vi "类型3一组自动测试.vi"(11 "测试值":u16) -> ()   [LabVIEW 2010]
uses:
  全局量/试验配置信息.vi
panel:
  out "D_IN_3":string[][](table) caption="表格"
  out "结束？":bool
  in  "同步_2":i32
  in  "同步_1":i32
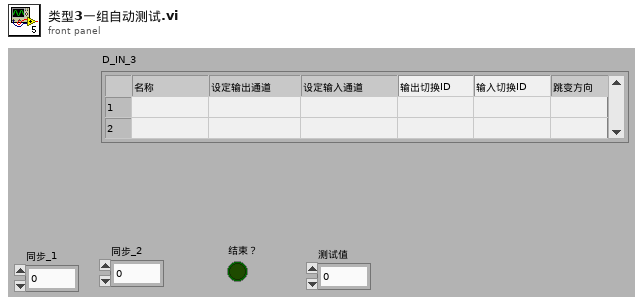
[diagram p1: front panel]
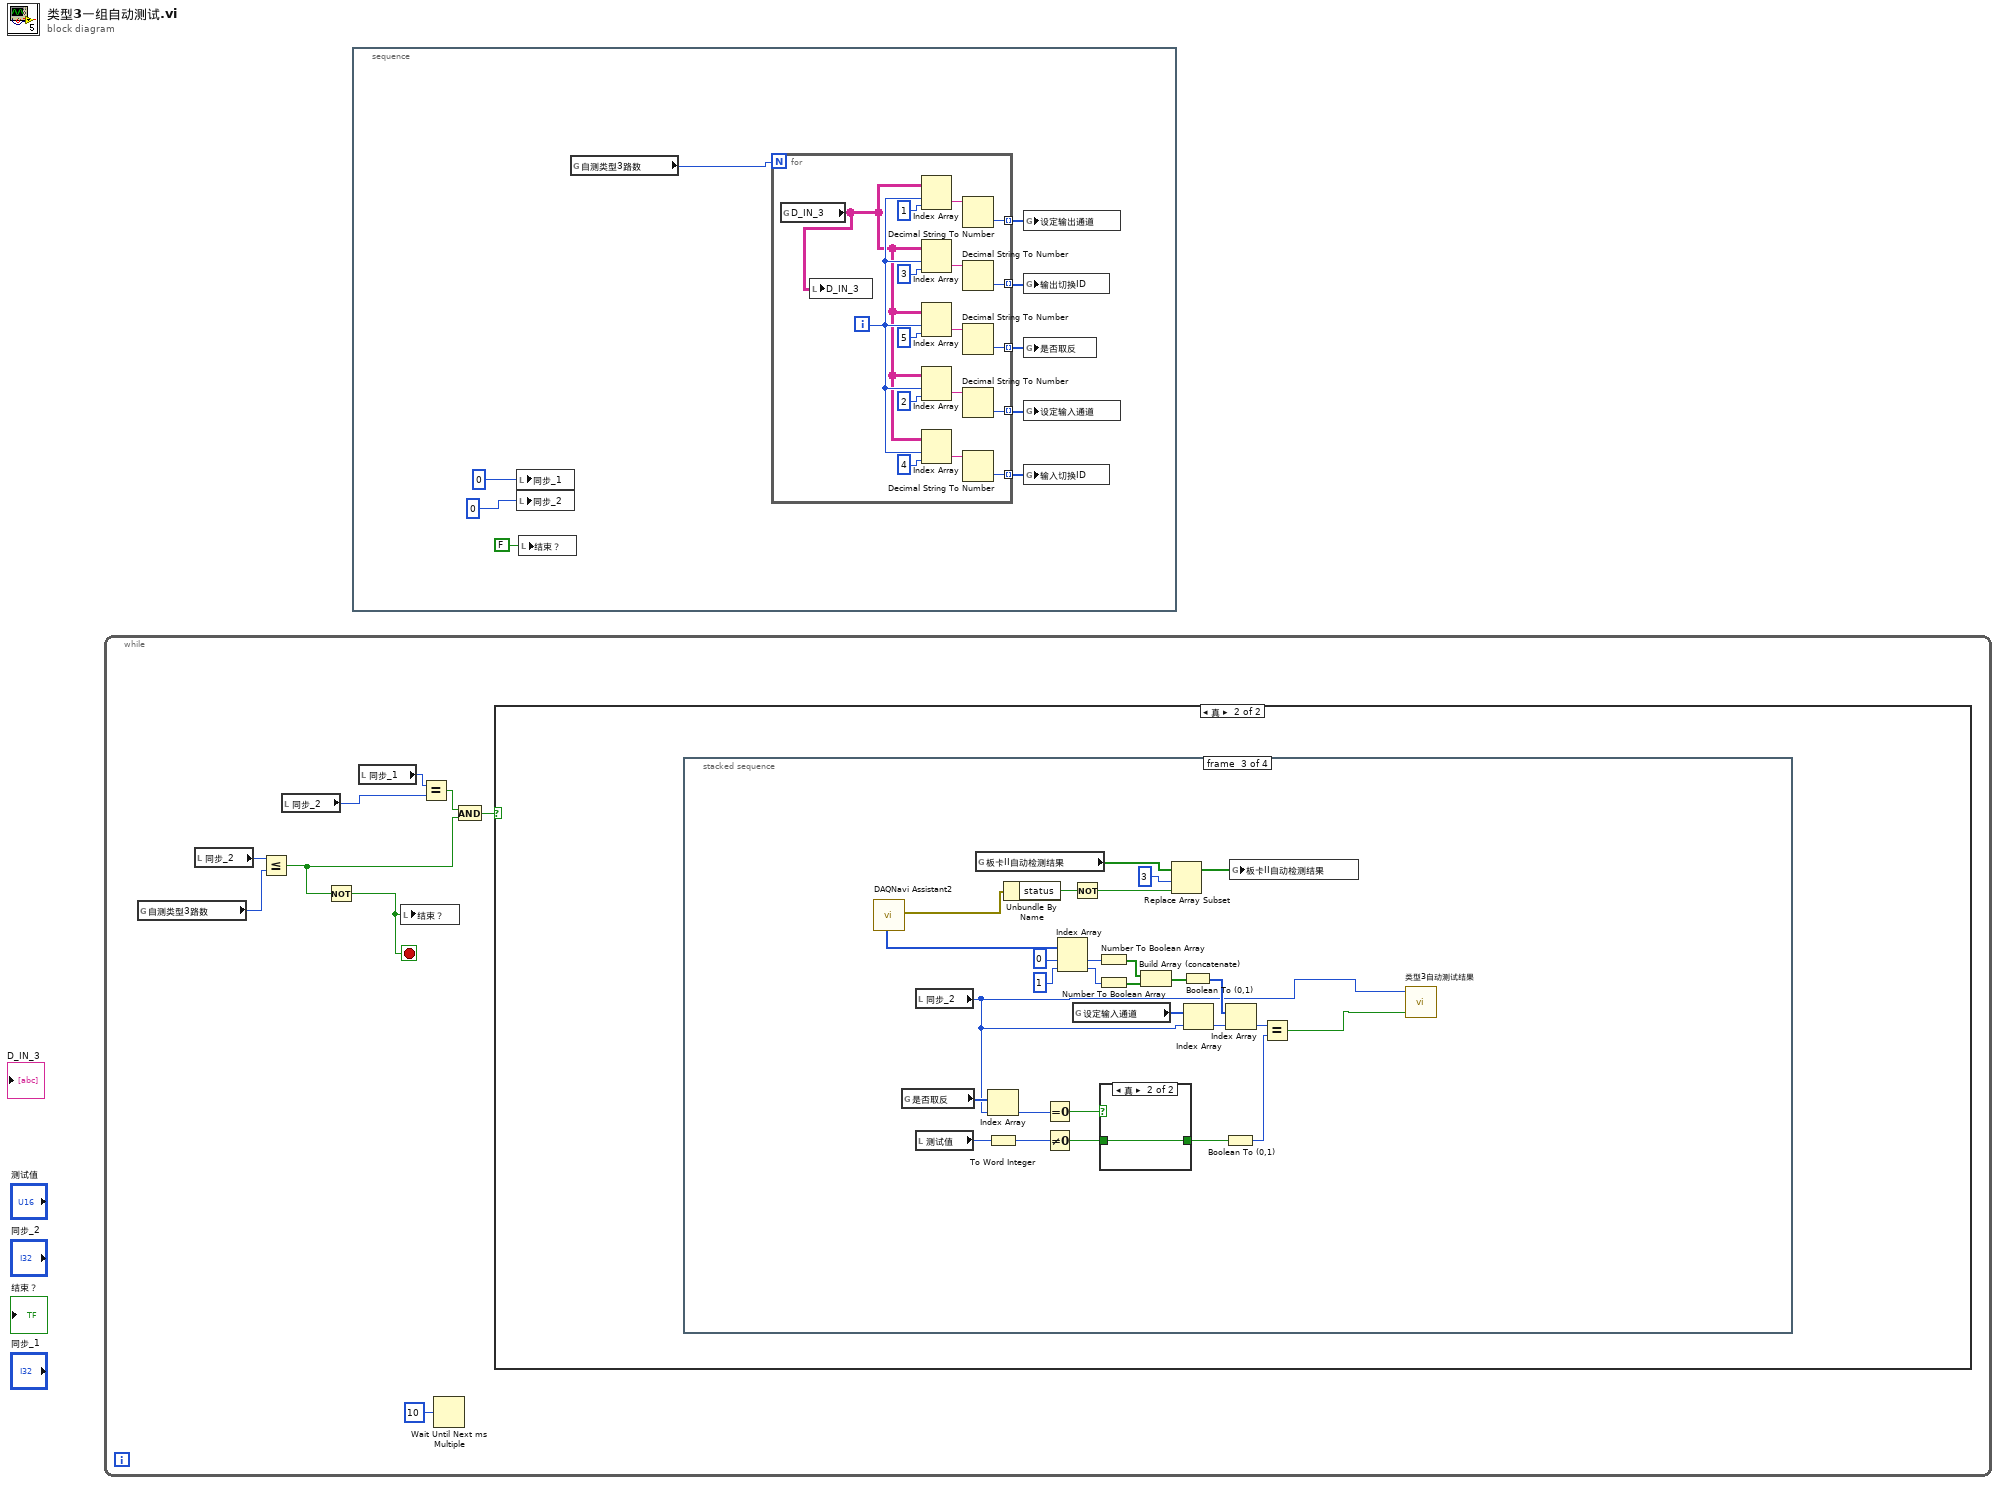
[diagram p0: block diagram]
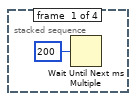
[diagram p3: hidden frame]
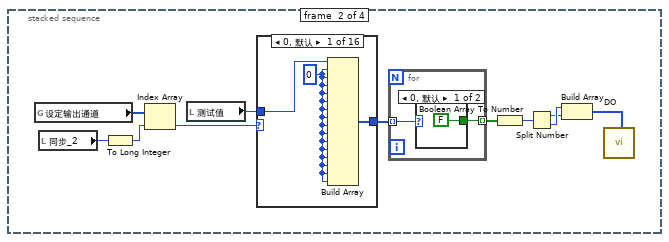
[diagram p4: hidden frame]
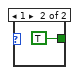
[diagram p5: hidden frame]
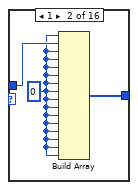
[diagram p6: hidden frame]
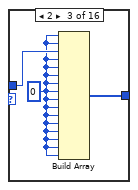
[diagram p7: hidden frame]
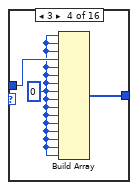
[diagram p8: hidden frame]
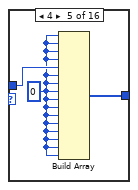
[diagram p9: hidden frame]
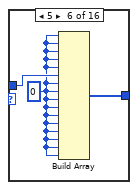
[diagram p10: hidden frame]
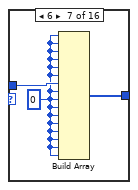
[diagram p11: hidden frame]
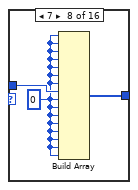
[diagram p12: hidden frame]
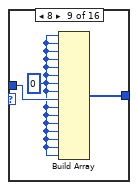
[diagram p13: hidden frame]
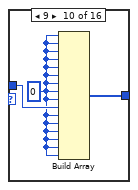
[diagram p14: hidden frame]
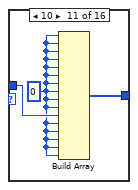
[diagram p15: hidden frame]
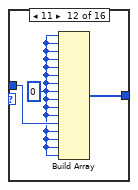
[diagram p16: hidden frame]
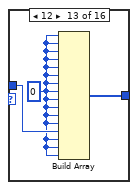
[diagram p17: hidden frame]
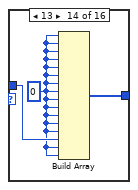
[diagram p18: hidden frame]
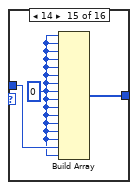
[diagram p19: hidden frame]
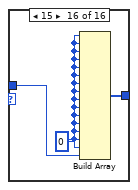
[diagram p20: hidden frame]
diagram:
  n1 = while {
    stop <- w2 stop-if-true
    n2 = global read "试验配置信息.vi" "自测类型3路数"() -> (w1:i32)
    n3 = local read "同步_2"() -> (w4:i32)
    n4 = Less Or Equal?(x=w4, y=w1) -> (x <= y?=w5:bool)
    n5 = local read "同步_2"() -> (w3:i32)
    n6 = Not(x=w5) -> (.not. x?=w2:bool)
    n7 = local read "同步_1"() -> (w8:i32)
    n8 = local write "结束？"(w2) -> ()
    n9 = Equal?(x=w8, y=w3) -> (x = y?=w6:bool)
    n10 = Wait Until Next ms Multiple(millisecond multiple=u32 10 ("毫秒倍数")) -> ()  [unwired: 1 out]
    n11 = And(x=w6, y=w5) -> (x .and. y?=w7:bool)
    n12 = case shown="真" w7 {
      frame False {
      }
      frame True {
        n13 = stacked-sequence {
          frame #0 {
            n14 = Wait Until Next ms Multiple(millisecond multiple=u32 200 ("毫秒倍数")) -> ()  [unwired: 1 out]
          }
          frame #1 {
            n15 = global read "试验配置信息.vi" "设定输出通道"() -> (w21:i32[])
            n16 = local read "同步_2"() -> (w11:i32)
            n17 = To Long Integer(number=w11) -> (32bit integer=w13:i32)
            n18 = Index Array(array=w21, index=w13) -> (element=w20:i32)
            n19 = local read "测试值"() -> (w12:u16)
            n20 = case shown="0, 默认" w20 {
              tunnel: w12 -> [w28 w31 w33 w36 w39 w42 w45 w48 w51 w54 w57 w60 w63 w66 w69 w72]
              tunnel: [w27 w30 w34 w37 w40 w43 w46 w49 w52 w55 w58 w61 w64 w67 w70 w73] -> w14
              frame 0, Default {
                w26 = 0 ("y")
                n21 = Build Array(w28, w26, w26, w26, w26, w26, w26, w26, w26, w26, w26, w26, w26, w26, w26, w26) -> (w27:i32[])
              }
              frame 1 {
                w29 = 0 ("y")
                n22 = Build Array(w29, w31, w29, w29, w29, w29, w29, w29, w29, w29, w29, w29, w29, w29, w29, w29) -> (w30:i32[])
              }
              frame 2 {
                w32 = 0 ("y")
                n23 = Build Array(w32, w32, w33, w32, w32, w32, w32, w32, w32, w32, w32, w32, w32, w32, w32, w32) -> (w34:i32[])
              }
              frame 3 {
                w35 = 0 ("y")
                n24 = Build Array(w35, w35, w35, w36, w35, w35, w35, w35, w35, w35, w35, w35, w35, w35, w35, w35) -> (w37:i32[])
              }
              frame 4 {
                w38 = 0 ("y")
                n25 = Build Array(w38, w38, w38, w38, w39, w38, w38, w38, w38, w38, w38, w38, w38, w38, w38, w38) -> (w40:i32[])
              }
              frame 5 {
                w41 = 0 ("y")
                n26 = Build Array(w41, w41, w41, w41, w41, w42, w41, w41, w41, w41, w41, w41, w41, w41, w41, w41) -> (w43:i32[])
              }
              frame 6 {
                w44 = 0 ("y")
                n27 = Build Array(w44, w44, w44, w44, w44, w44, w45, w44, w44, w44, w44, w44, w44, w44, w44, w44) -> (w46:i32[])
              }
              frame 7 {
                w47 = 0 ("y")
                n28 = Build Array(w47, w47, w47, w47, w47, w47, w47, w48, w47, w47, w47, w47, w47, w47, w47, w47) -> (w49:i32[])
              }
              frame 8 {
                w50 = 0 ("y")
                n29 = Build Array(w50, w50, w50, w50, w50, w50, w50, w50, w51, w50, w50, w50, w50, w50, w50, w50) -> (w52:i32[])
              }
              frame 9 {
                w53 = 0 ("y")
                n30 = Build Array(w53, w53, w53, w53, w53, w53, w53, w53, w53, w54, w53, w53, w53, w53, w53, w53) -> (w55:i32[])
              }
              frame 10 {
                w56 = 0 ("y")
                n31 = Build Array(w56, w56, w56, w56, w56, w56, w56, w56, w56, w56, w57, w56, w56, w56, w56, w56) -> (w58:i32[])
              }
              frame 11 {
                w59 = 0 ("y")
                n32 = Build Array(w59, w59, w59, w59, w59, w59, w59, w59, w59, w59, w59, w60, w59, w59, w59, w59) -> (w61:i32[])
              }
              frame 12 {
                w62 = 0 ("y")
                n33 = Build Array(w62, w62, w62, w62, w62, w62, w62, w62, w62, w62, w62, w62, w63, w62, w62, w62) -> (w64:i32[])
              }
              frame 13 {
                w65 = 0 ("y")
                n34 = Build Array(w65, w65, w65, w65, w65, w65, w65, w65, w65, w65, w65, w65, w65, w66, w65, w65) -> (w67:i32[])
              }
              frame 14 {
                w68 = 0 ("y")
                n35 = Build Array(w68, w68, w68, w68, w68, w68, w68, w68, w68, w68, w68, w68, w68, w68, w69, w68) -> (w70:i32[])
              }
              frame 15 {
                w71 = 0 ("y")
                n36 = Build Array(w71, w71, w71, w71, w71, w71, w71, w71, w71, w71, w71, w71, w71, w71, w71, w72) -> (w73:i32[])
              }
            }
            n37 = for {
              tunnel: w14 -> [w23] mode=indexing
              tunnel: [w22] -> w19 mode=indexing
              n38 = case shown="0, 默认" w23 {
                tunnel: [FALSE TRUE] -> w22
                frame 0, Default {
                }
                frame 1 {
                }
              }
            }
            n39 = Boolean Array To Number ("布尔数组至数值转换")(Boolean array=w19) -> (number=w18:u16)
            n40 = Split Number(x=w18) -> (hi(x)=w15:u8, lo(x)=w16:u8)
            n41 = Build Array(w16, w15) -> (w17:u8[])
            n42 = call "DO"("dataIn(U8Array)"=w17) -> ()  [unwired: 2 in, 17 out]
          }
          frame #2 {
            n43 = call "DAQNavi Assistant2"() -> ("error out"=w81:errorcluster, "dataOut(U8Array)"=w100:u8[])  [unwired: 2 in, 16 out]
            n44 = global read "试验配置信息.vi" "是否取反"() -> (w98:i32[])
            n45 = local read "同步_2"() -> (w77:i32)
            n46 = local read "测试值"() -> (w101:u16)
            n47 = global read "试验配置信息.vi" "板卡II自动检测结果"() -> (w82:bool[])
            n48 = Index Array(array=w98, index=w77) -> (element=w97:i32)
            n49 = To Word Integer ("转换为双字节整型")(number=w101) -> (16bit integer=w99:i16)
            n50 = Unbundle By Name(w81) -> ("status"=w80:bool)
            n51 = Equal To 0?(x=w97) -> (x = 0?=w96:bool)
            n52 = Not Equal To 0?(x=w99) -> (x != 0?=w78:bool)
            n53 = Index Array(array=w100, index #1=0 ("索引"), index #2=1 ("索引")) -> (element #1=w90:u8, element #2=w91:u8)
            n54 = Not(x=w80) -> (.not. x?=w79:bool)
            n55 = global read "试验配置信息.vi" "设定输入通道"() -> (w85:i32[])
            n56 = Number To Boolean Array(number=w90) -> (Boolean array=w86:bool[])
            n57 = Number To Boolean Array(number=w91) -> (Boolean array=w87:bool[])
            n58 = case shown="真" w96 {
              tunnel: w78 -> [w103 w104]
              tunnel: [w102 w104] -> w95
              frame False {
                n59 = Not(x=w103) -> (.not. x?=w102:bool)
              }
              frame True {
              }
            }
            n60 = Build Array (concatenate)(w86, w87) -> (w92:bool[])
            n61 = Replace Array Subset(array=w82, new element=w79, index=3 ("索引")) -> (w83:bool[])
            n62 = Boolean To (0,1) ("布尔值至(0,1)转换")(Boolean=w92) -> (0, 1=w93:i16[])
            n63 = Index Array(array=w85, index=w77) -> (element=w94:i32)
            n64 = Boolean To (0,1)(Boolean=w95) -> (0, 1=w75:i16)
            n65 = Index Array(array=w93, index=w94) -> (element=w76:i16)
            n66 = global write "试验配置信息.vi" "板卡II自动检测结果"(w83) -> ()
            n67 = Equal?(x=w76, y=w75) -> (x = y?=w74:bool)
            n68 = call "类型3自动测试结果.vi"("合格?"=w74, "第几组"=w77) -> ()  [unwired: 10 in]
          }
          frame #3 {
            n69 = local read "同步_1"() -> (w106:i32)
            n70 = local read "同步_2"() -> (w108:i32)
            n71 = Increment(x=w106) -> (x+1=w105:i32)
            n72 = Increment(x=w108) -> (x+1=w107:i32)
            n73 = local write "同步_2"(w107) -> ()
            n74 = local write "同步_1"(w105) -> ()
          }
        }
      }
    }
  }
  n75 = stacked-sequence {
    frame #0 {
      n76 = local write "同步_1"(0 ("同步_1")) -> ()
      n77 = local write "同步_2"(0 ("同步_1")) -> ()
      n78 = local write "结束？"(FALSE ("结束？")) -> ()
      n79 = global read "试验配置信息.vi" "自测类型3路数"() -> (w109:i32)
      n80 = for {
        N: w109 -> [_]
        tunnel: [w132] -> w110 mode=indexing
        tunnel: [w129] -> w111 mode=indexing
        tunnel: [w126] -> w112 mode=indexing
        tunnel: [w123] -> w113 mode=indexing
        tunnel: [w119] -> w114 mode=indexing
        i -> [w121]
        n81 = global read "试验配置信息.vi" "D_IN_3"() -> (w118:string[][])
        n82 = local write "D_IN_3"(w118) -> ()
        n83 = Index Array(array=w118, index (row)=w121, index (col)=1 ("禁用的索引 (列)")) -> (element=w131:string)
        n84 = Index Array(array=w118, index (row)=w121, index (col)=3 ("禁用的索引 (列)")) -> (element=w127:string)
        n85 = Index Array(array=w118, index (row)=w121, index (col)=5 ("禁用的索引 (列)")) -> (element=w120:string)
        n86 = Index Array(array=w118, index (row)=w121, index (col)=2 ("禁用的索引 (列)")) -> (element=w133:string)
        n87 = Index Array(array=w118, index (row)=w121, index (col)=4 ("禁用的索引 (列)")) -> (element=w124:string)
        n88 = Decimal String To Number(string=w131) -> (number=w129:i32)  [unwired: 2 in, 1 out]
        n89 = Decimal String To Number(string=w127) -> (number=w126:i32)  [unwired: 2 in, 1 out]
        n90 = Decimal String To Number(string=w120) -> (number=w119:i32)  [unwired: 2 in, 1 out]
        n91 = Decimal String To Number(string=w133) -> (number=w132:i32)  [unwired: 2 in, 1 out]
        n92 = Decimal String To Number(string=w124) -> (number=w123:i32)  [unwired: 2 in, 1 out]
      }
      n93 = global write "试验配置信息.vi" "设定输出通道"(w111) -> ()
      n94 = global write "试验配置信息.vi" "输出切换ID"(w112) -> ()
      n95 = global write "试验配置信息.vi" "是否取反"(w114) -> ()
      n96 = global write "试验配置信息.vi" "设定输入通道"(w110) -> ()
      n97 = global write "试验配置信息.vi" "输入切换ID"(w113) -> ()
    }
  }
